vi "Brute Force Dark Current Primary Logic Body.vi"(0 "Barcodes in":string[](array[string]), 1 "stop":bool, 2 "Pins In":refnum<k21>[](array[refnum]), 5 "VISA Refnum in":refnum<visa-resource-name>, 6 "Number of Tubes":i32, 7 "Channel #":i32) -> (10 "Actual Voltage Level (V)":dbl format="%#_13g", 11 "Individual Tube Current (Nano Amps)":dbl[](array[numeric]), 12 "Actual Current Limit (nA)":dbl format="%#_13g", 13 "Mesurnment Iteration":i32, 14 "Power Supply Trip":bool, 16 "Pins Out":refnum<k21>[](array[refnum]), 19 "Failed Tubes":string[](array[string]))   [LabVIEW 2020]
uses:
  SUB VI Dark Current Test Files 2018 For Drop Box/Program Files (x86)/National Instruments/LabVIEW 2020/instr.lib/CAEN PSM/CAEN PSM.lvlib
panel:
  out "error out":errorcluster
  in  "First Tube #":i32
  out "BoardHandle out":T1
  # "Pin in"
  # "Pin out"
  # "No pin"
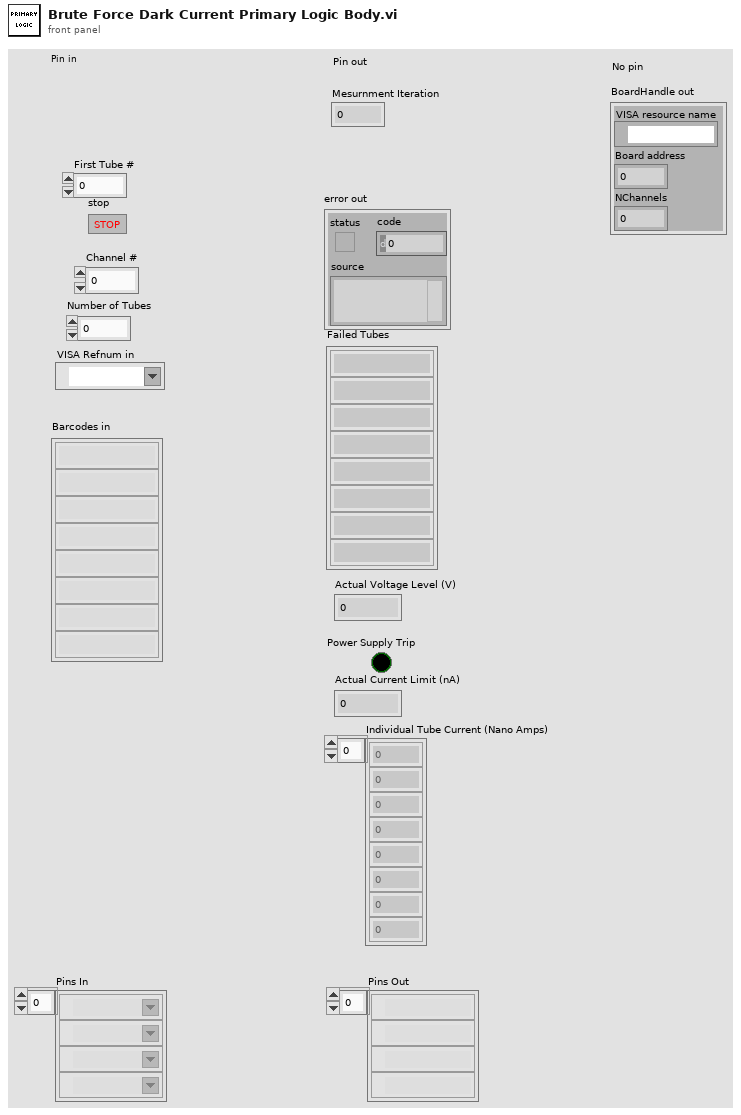
[diagram p1: front panel]
types:
  T1 = cluster{"VISA resource name":refnum<visa-resource-name>, "Board address":u8, "NChannels":u8}
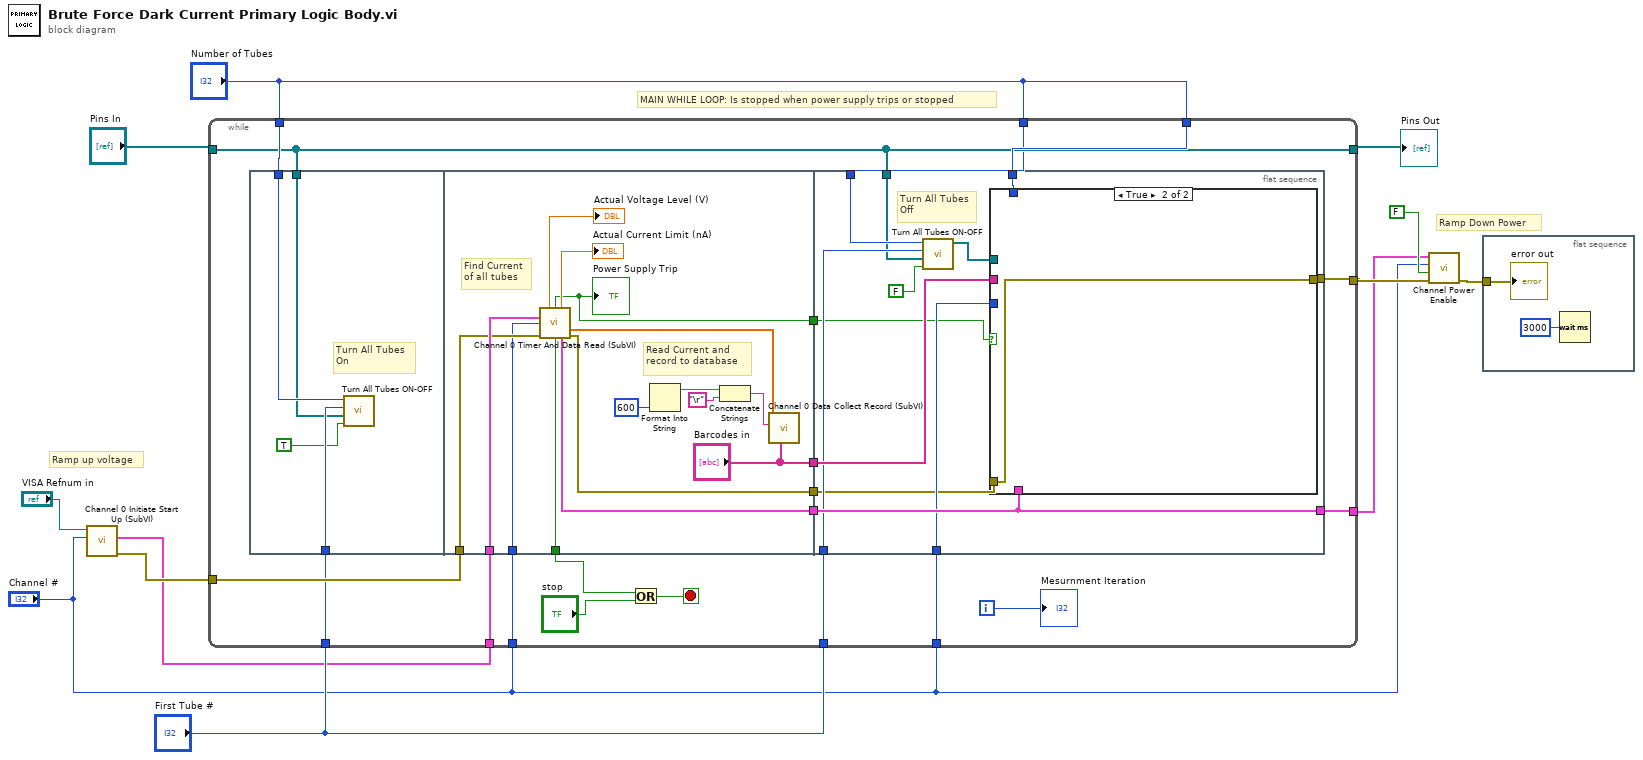
[diagram p0: block diagram]
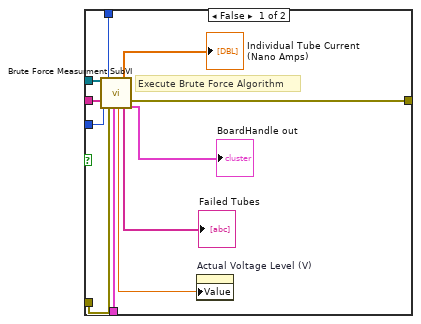
[diagram p2: hidden frame]
diagram:
  # "Ramp Down Power"
  # "MAIN WHILE LOOP: Is stopped when power supply trips or stopped"
  # "Ramp up voltage"
  n1 = call "Channel 0 Initiate Start Up (SubVI).vi"("Channel # in"="Channel #", "VISA Refnum in"="VISA Refnum in") -> ("error out"=w7:errorcluster, "BoardHandle out"=w6:T1)  [unwired: 8 in]
  n2 = while {
    tunnel: "Number of Tubes" -> [w32]
    tunnel: "First Tube #" -> [w31]
    tunnel: "Number of Tubes" -> [w14]
    tunnel: "Channel #" -> [w30]
    tunnel: w6 -> [w29]
    tunnel: "Number of Tubes" -> [w28]
    tunnel: w7 -> [w24]
    tunnel: "First Tube #" -> [w20]
    tunnel: [w18] -> w9
    tunnel: [w17] -> w11
    tunnel: "Pins In" -> [w15]
    tunnel: "Channel #" -> [w16]
    tunnel: [w15] -> w2
    i -> [w21]
    stop <- w22 stop-if-true
    n3 = flat-sequence {
      tunnel: w28 -> [w36]
      tunnel: w20 -> [w35]
      tunnel: w15 -> [w33]
      tunnel: w30 -> [w39]
      tunnel: w29 -> [w42]
      tunnel: [w46] -> w27
      tunnel: [w44] -> w26
      tunnel: ["Barcodes in"] -> w25
      tunnel: w24 -> [w41]
      tunnel: [w37] -> w23
      tunnel: [w37] -> w13
      tunnel: w32 -> [w61]
      tunnel: w25 -> [w62]
      tunnel: w26 -> [w60]
      tunnel: w27 -> [w54]
      tunnel: w14 -> [w59]
      tunnel: w31 -> [w58]
      tunnel: [w60] -> w18
      tunnel: [w53] -> w17
      tunnel: w16 -> [w56]
      tunnel: w15 -> [w55]
      tunnel: w13 -> [w51]
      frame #0 {
        # "Turn All Tubes \nOn"
        n4 = call "Turn All Tubes ON-OFF.vi"("Activate: 1\nDeactivate: 0"=TRUE, "Pins In"=w33, "First Tube #"=w35, "Last Tube #"=w36) -> ()  [unwired: 7 in, 1 out]
      }
      frame #1 {
        # "Find Current\nof all tubes"
        # "Read Current and  record to database"
        n5 = call "Channel 0 Timer And Data Read (SubVI).vi"("BoardHandle in"=w42, "Channel # in"=w39, "error in (no error)"=w41) -> ("Actual Voltage Level (V)"=→"Actual Voltage Level (V)":dbl, "Power Supply Trip"=w37:bool, "Actual Current Limit (nA)"=→"Actual Current Limit (nA)":dbl, "Array"=w45:dbl[], "BoardHandle out 2"=w44:T1, "error out"=w46:errorcluster)  [unwired: 7 in]
        "Power Supply Trip" <- w37
        n6 = Format Into String(600 ("input 1")) -> (resulting string=w49:string)  [unwired: 3 in, 1 out]
        n7 = Concatenate Strings(w49, "\r") -> (w50:string)
        n8 = call "Channel 0 Data Collect Record (SubVI).vi"("Barcodes"="Barcodes in", "Array"=w45, "String"=w50) -> ()  [unwired: 9 in]
      }
      frame #2 {
        # "Turn All Tubes\nOff"
        n9 = call "Turn All Tubes ON-OFF.vi"("Activate: 1\nDeactivate: 0"=FALSE ("Activate: 1\nDeactivate: 0"), "Pins In"=w55, "First Tube #"=w58, "Last Tube #"=w59) -> ("Pins Out"=w52:refnum<k21>[])  [unwired: 7 in]
        n10 = case shown="True" w51 {
          tunnel: w62 -> [w73 _]
          tunnel: w61 -> [w72 _]
          tunnel: w60 -> [w71 _]
          tunnel: w56 -> [w66 _]
          tunnel: w54 -> [w65 w74]
          tunnel: [w64 w74] -> w53
          tunnel: w52 -> [w63 _]
          frame False {
            # "Execute Brute Force Algorithm"
            n11 = call "Brute Force Measurment SubVI.vi"("Pins In"=w63, "Barcodes in"=w73, "Channel # in"=w66, "Last Tube #"=w72, "error in (no error)"=w65, "BoardHandle in"=w71) -> ("Actual Voltage Level (V) 2"=w70:dbl, "Individual Tube Current (Nano Amps)"=→"Individual Tube Current (Nano Amps)":dbl[], "Failed Tubes"=→"Failed Tubes":string[], "error out"=w64:errorcluster, "BoardHandle out"=→"BoardHandle out":T1)  [unwired: 8 in, 1 out]
            n12 = property on="Actual Voltage Level (V)" class="DigNum (strict)"("Value"=w70) -> ()  [unwired: 2 in, 2 out]
          }
          frame True {
          }
        }
      }
    }
    n13 = Or(x=w23, y="stop") -> (x .or. y?=w22:bool)
    "Mesurnment Iteration" <- w21
  }
  "Pins Out" <- w2
  n14 = call "Channel Power Enable.vi"("error in (no error)"=w11, "Enable (OFF)"=FALSE, "Channel (0)"="Channel #", "BoardHandle"=w9) -> ("error out"=w1:errorcluster)  [unwired: 6 in, 1 out]
  n15 = flat-sequence {
    tunnel: w1 -> [w76]
    frame #0 {
      n16 = Wait (ms)(milliseconds to wait=u32 3000) -> ()  [unwired: 1 out]
      "error out" <- w76
    }
  }
